vi "ArrayDevScan.vi"(6 "CurPointInd":i32, 8 "error in":errorcluster caption="entrée d'erreur (pas d'erreur)", 9 "IndCourbe":i64, 10 "DevID":i32, 11 "Experiment.lvclass In":refnum<class "Experiment.lvclass">) -> (0 "error out":errorcluster caption="sortie d'erreur", 1 "ArrNomDon":string[](array[string])=["RTêta;", "X&Y;"], 2 "HeaderPar":string, 3 "ArrVarParsOut":string[][](array[string]), 4 "ArrScan list":string[](array[string]), 5 "ArrVarPar list":string[](array[string]))   [LabVIEW 2019, in "Experiment.lvclass"]
uses:
  Experiment.lvclass
  Experiment.lvclass/Experiment.ctl
  DevicesClass/BaseDevice/BaseDevice.lvclass
panel:
  in  "VarParams":string[][](array[string])
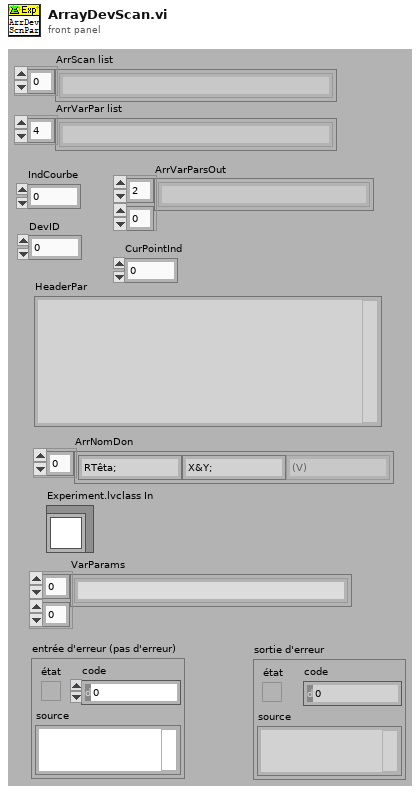
[diagram p1: front panel]
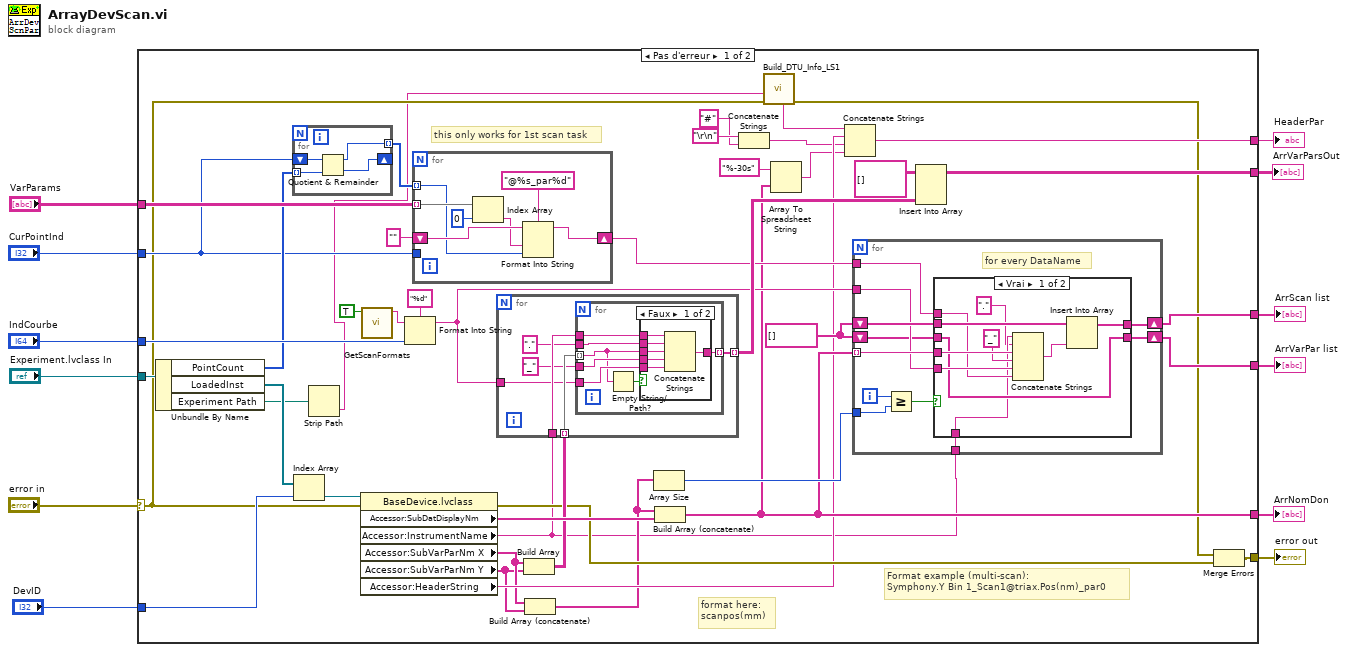
[diagram p0: block diagram]
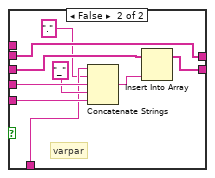
[diagram p3: hidden frame]
diagram:
  n1 = case shown="Pas d'erreur" "error in" {
    selector: "error in" -> [w19 w117]
    tunnel: [w55 w117] -> w11
    tunnel: [w29 _] -> w10
    tunnel: "Experiment.lvclass In" -> [w42 _]
    tunnel: "IndCourbe" -> [w54 _]
    tunnel: [w53 _] -> w7
    tunnel: "DevID" -> [w52 _]
    tunnel: [w38 _] -> w5
    tunnel: [w37 _] -> w4
    tunnel: "CurPointInd" -> [w24 _]
    tunnel: "VarParams" -> [w35 _]
    tunnel: [w26 _] -> w1
    frame No Error {
      w36 = string[] []
      # "this only works for 1st scan task"
      # "Format example (multi-scan):\nSymphony.Y Bin 1_Scan1@triax.Pos(nm)_par0"
      # "format here:\nscanpos(mm)"
      n2 = Unbundle By Name(w42) -> ("PointCount"=w25:i32[], "LoadedInst"=w43:refnum<class "BaseDevice.lvclass">[], "Experiment Path"=w14:path)
      n3 = for {
        tunnel: w25 -> [w78] mode=indexing
        shift-right: [w77] -> _
        shift-left: w24 -> [w79]
        tunnel: [w76] -> w23 mode=indexing
        n4 = Quotient & Remainder(x=w79, y=w78) -> (x-y*floor(x/y)=w76:i32, floor(x/y)=w77:i32)
      }
      n5 = Index Array(array=w43, index=w52) -> (element=w49:refnum<class "BaseDevice.lvclass">)
      n6 = Strip Path(path=w14) -> (name=w13:string)  [unwired: 1 out]
      n7 = property class="BaseDevice.lvclass"(reference=w49, error in=w19) -> (error out=w41:errorcluster, "Accessor:SubDatDisplayNm"=w45:string[], "Accessor:InstrumentName"=w15:string, "Accessor:SubVarParNm X"=w18:string[], "Accessor:SubVarParNm Y"=w17:string[], "Accessor:HeaderString"=w28:string)  [unwired: 1 out]
      n8 = call "GetScanFormats.vi"("Scan(T)"=TRUE) -> ("Prefixe"=w48:string)  [unwired: 8 in, 2 out]
      n9 = Format Into String(format string="%d" ("chaîne de format"), initial string=w48, w54) -> (resulting string=w39:string)  [unwired: 1 in, 1 out]
      n10 = for {
        tunnel: w35 -> [w86] mode=indexing
        tunnel: w24 -> [_]
        shift-right: [w83] -> w34
        shift-left: "" -> [w82]
        tunnel: w23 -> [w80] mode=indexing
        n11 = Index Array(array=w86, index=0 ("indice")) -> (element=w81:string)
        n12 = Format Into String(format string="@%s_par%d" ("chaîne de format"), initial string=w82, w81, w80) -> (resulting string=w83:string)  [unwired: 1 in, 1 out]
      }
      n13 = Build Array(w18, w17) -> (w44:string[][])
      n14 = for {
        tunnel: [w61] -> w51 mode=indexing
        tunnel: w15 -> [w60]
        tunnel: w44 -> [w59] mode=indexing
        tunnel: w39 -> [w58]
        n15 = for {
          tunnel: w59 -> [w62] mode=indexing
          tunnel: "." ("chaîne") -> [w68]
          tunnel: [w67] -> w61 mode=indexing
          tunnel: w60 -> [w66]
          tunnel: "_" ("chaîne") -> [w64]
          tunnel: w58 -> [w65]
          n16 = Empty String/Path?(string/path=w62) -> (empty?=w63:bool)
          n17 = case shown="Faux" w63 {
            tunnel: w62 -> [w74 w75]
            tunnel: w68 -> [w73 _]
            tunnel: [w72 w75] -> w67
            tunnel: w66 -> [w71 _]
            tunnel: w65 -> [w70 _]
            tunnel: w64 -> [w69 _]
            frame False {
              n18 = Concatenate Strings(w71, w73, w74, w69, w70) -> (w72:string)
            }
            frame True {
            }
          }
        }
      }
      n19 = Build Array (concatenate)(w18, w17) -> (w16:string[])
      n20 = Array Size(array=w16) -> (size(s)=w40:i32)
      n21 = Build Array (concatenate)(w16, w45) -> (w29:string[])
      n22 = Concatenate Strings("\r\n", "#" ("chaîne")) -> (w21:string)
      n23 = call "Build_DTU_Info_LS1.vi"("error in"=w19, "Experiment Path"=w13) -> ("error out"=w20:errorcluster, "DTU_HdrStr"=w22:string)  [unwired: 3 in, 5 out]
      n24 = Array To Spreadsheet String(array=w29, 3:"%-30s" ("format string")) -> (spreadsheet string=w27:string)  [unwired: 1 in]
      n25 = Concatenate Strings(w22, w28, w21, w27) -> (w26:string)
      n26 = for {
        tunnel: w39 -> [w94]
        tunnel: w29 -> [w95] mode=indexing
        shift-right: [w96] -> w37
        shift-left: w36 -> [w97]
        tunnel: w40 -> [w93]
        shift-right: [w89] -> w38
        shift-left: w36 -> [w90]
        tunnel: w34 -> [w88]
        tunnel: w15 -> [w87]
        i -> [w92]
        # "for every DataName"
        n27 = Greater Or Equal?(x=w92, y=w93) -> (x >= y?=w91:bool)
        n28 = case shown="Vrai" w91 {
          tunnel: w97 -> [w107 w110]
          tunnel: [w106 w110] -> w96
          tunnel: w95 -> [w105 w116]
          tunnel: w94 -> [w104 w115]
          tunnel: w90 -> [w101 w112]
          tunnel: [w101 w111] -> w89
          tunnel: w88 -> [w100 _]
          tunnel: w87 -> [w99 w109]
          frame True {
            n29 = Concatenate Strings(w99, "." ("chaîne"), w105, "_" ("chaîne"), w104, w100) -> (w103:string)
            n30 = Insert Into Array(array=w107, new element=w103) -> (w106:string[])  [unwired: 1 in]
          }
          frame False {
            # "varpar"
            n31 = Concatenate Strings(w109, "." ("chaîne"), w116, "_" ("chaîne"), w115) -> (w114:string)
            n32 = Insert Into Array(array=w112, new element=w114) -> (w111:string[])  [unwired: 1 in]
          }
        }
      }
      n33 = Insert Into Array(array=string[][] [] ("VarParsOut"), new element=w51) -> (w53:string[][])  [unwired: 2 in]
      n34 = Merge Errors(w20, w41) -> (w55:errorcluster)
    }
    frame Error {
    }
  }
  "error out" <- w11
  "HeaderPar" <- w1
  "ArrNomDon" <- w10
  "ArrVarParsOut" <- w7
  "ArrScan list" <- w4
  "ArrVarPar list" <- w5
